vi "KH TURCK ETHERNETIP RFID Busyfinished1.vi"(6 "NoOfModules":i32, 7 "Function":string, 10 "IndexOfModule":i32, 11 "Busy":bool) -> (1 "Busy finished":bool, 3 "Busy OUT":bool)   [LabVIEW 2021]
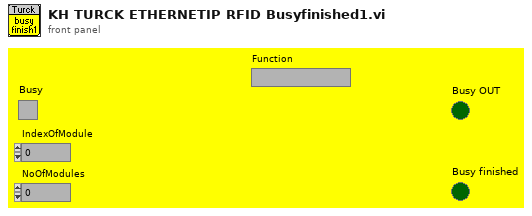
[diagram p1: front panel]
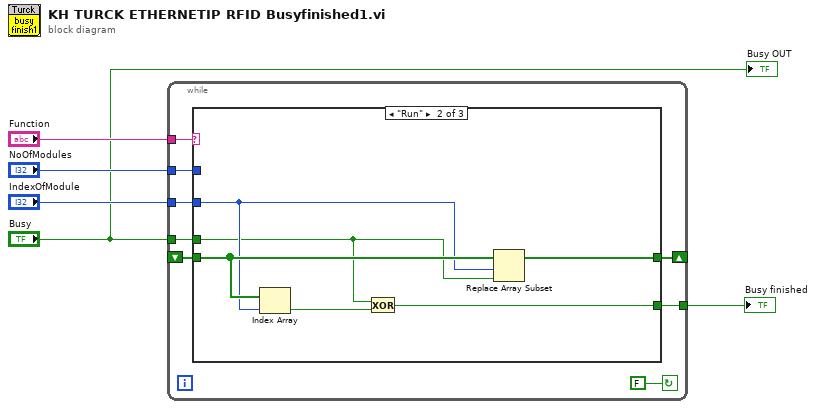
[diagram p0: block diagram]
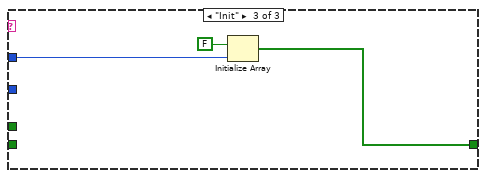
[diagram p3: hidden frame]
diagram:
  n1 = while {
    tunnel: "Function" -> [w12]
    shift-right: [w10] -> _
    shift-left: _ -> [w9]
    tunnel: "NoOfModules" -> [w11]
    tunnel: "IndexOfModule" -> [w8]
    tunnel: "Busy" -> [w7]
    tunnel: [w6] -> w1
    stop <- FALSE continue-if-true
    n2 = case shown="\"Run\"" w12 {
      tunnel: w11 -> [_ _ w23]
      tunnel: [w14 w16 w21] -> w10
      tunnel: w9 -> [w14 w19 _]
      tunnel: w8 -> [_ w18 _]
      tunnel: w7 -> [_ w17 _]
      tunnel: [_ w15 _] -> w6
      frame Default {
      }
      frame "Run" {
        n3 = Index Array(array=w19, index=w18) -> (element=w20:bool)
        n4 = Exclusive Or(1:w20, 2:w17) -> (0:w15:bool)
        n5 = Replace Array Subset(array=w19, new element=w17, index=w18) -> (w16:bool[])
      }
      frame "Init" {
        n6 = Initialize Array(FALSE, w23) -> (w21:bool[])
      }
    }
  }
  "Busy finished" <- w1
  "Busy OUT" <- "Busy"
